vi "Verify Remote VIPM Repository.vi"(8 "error in (no error)":errorcluster, 11 "Artifactory.VIPM in":refnum<class "Artifactory.VIPM.lvclass">) -> (0 "error out":errorcluster, 1 "Read Permission":bool, 2 "Repository exists":bool, 3 "Artifactory.VIPM out":refnum<class "Artifactory.VIPM.lvclass">)   [LabVIEW 2021, in "Artifactory.VIPM.lvclass"]
uses:
  Artifactory.VIPM.lvclass
  C:/Repositories/LVOS/Artifactory/lv-src/Artifactory/Artifactory.lvclass
  Artifactory.VIPM.lvclass/Artifactory.VIPM.ctl
  Artifactory/Artifactory.lvclass
  C:/Repositories/LVOS/Artifactory/lv-src/Artifactory.VIPM/Artifactory.VIPM.lvclass
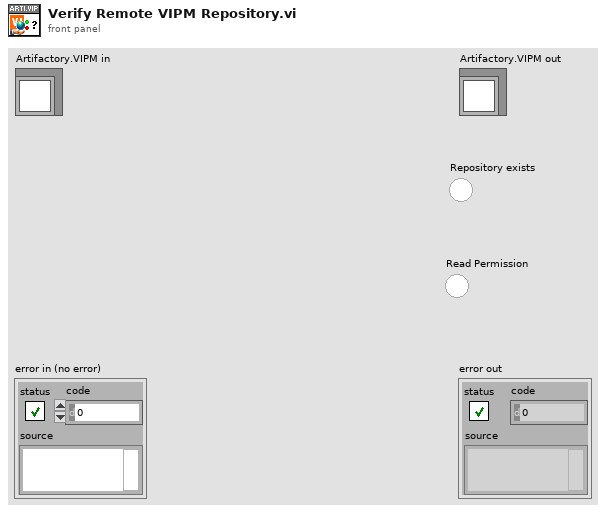
[diagram p1: front panel]
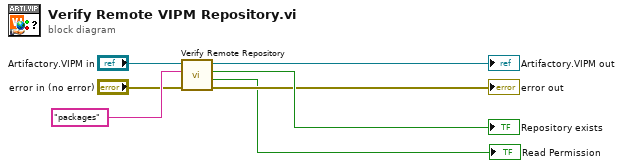
[diagram p0: block diagram]
diagram:
  n1 = call "Verify Remote Repository.vi"("error in (no error)"="error in (no error)", "folder (root)"="packages", "Artifactory in"="Artifactory.VIPM in") -> ("error out"=→"error out":errorcluster, "Read Permissions"=→"Read Permission":bool, "Repository exists"=→"Repository exists":bool, "Artifactory out"=→"Artifactory.VIPM out":refnum<class "Artifactory.VIPM.lvclass">)  [unwired: 5 in]
